vi "CloseAllDevices.vi"(0 "Signal Generator":refnum<class "Signal Generation.lvclass">, 5 "Scope":refnum<class "Scope.lvclass">, 7 "Meter":refnum<class "Meter.lvclass">, 9 "Switch":refnum<class "Switch.lvclass">, 11 "error in (no error)":errorcluster) -> (15 "error out":errorcluster)   [LabVIEW 2011]
doc: "This function does not have any inputs or outputs other than the error clusters. It uses the DSSP class global variables to call the Close VIs for each DSSP class that is being used. Each DSSP Close VI then takes care of closing the resource session for the specific instrument."
uses:
  DSSP Modules/Output Classes/Signal Generation/Signal Generation.lvclass
  DSSP Modules/Input Classes/Scope/Scope.lvclass
  DSSP Modules/Input Classes/Meter/Meter.lvclass
  DSSP Modules/Output Classes/Switch/Switch.lvclass
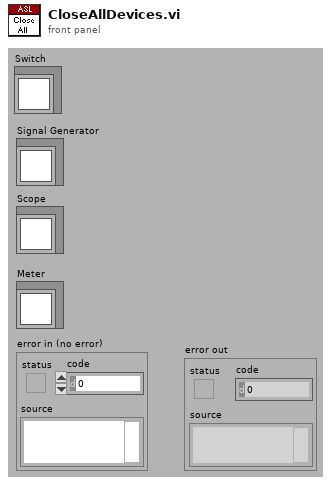
[diagram p1: front panel]
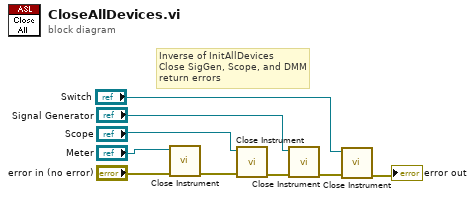
[diagram p0: block diagram]
diagram:
  # "Inverse of InitAllDevices\nClose SigGen, Scope, and DMM\nreturn errors"
  n1 = call-dynamic "Close Instrument.vi"("error in (no error)"="error in (no error)", "DSSP.lvclass in"="Meter") -> ("error out"=w8:errorcluster)  [unwired: 9 out]
  n2 = call-dynamic "Close Instrument.vi"("error in (no error)"=w8, "DSSP.lvclass in"="Scope") -> ("error out"=w7:errorcluster)  [unwired: 9 out]
  n3 = call-dynamic "Close Instrument.vi"("error in (no error)"=w7, "DSSP.lvclass in"="Signal Generator") -> ("error out"=w3:errorcluster)  [unwired: 9 out]
  n4 = call-dynamic "Close Instrument.vi"("error in (no error)"=w3, "DSSP.lvclass in"="Switch") -> ("error out"=→"error out":errorcluster)  [unwired: 9 out]
